vi "Prepare_TTL_activation_sequence.vi"(5 "Conditions presets array":T1 {"Specifier(s)"."Validity criteria(s)"."Validity value" min=0.0 step=0.1 format="%.2g"; "Specifier(s)"."Value" step=1.0 format="%#.2g"}, 7 "IO parameters.IO inversion config.":u16, 8 "Error In":errorcluster, 10 "Rules (conditions) became FALSE":bool[](array[boolean])=[FALSE, FALSE, FALSE, FALSE], 11 "Rules (conditions) became TRUE":bool[](array[boolean])=[FALSE, FALSE, FALSE, FALSE]) -> (0 "Error Out":errorcluster, 3 "TTL command(s) out":cluster{"Numeric":dbl, "String":string}[](array[cluster]))   [LabVIEW 2018, in "TTL IO.lvlib"]
uses:
  TTL IO.lvlib
  SubVi's/Controls/CTL_Conditions_Array.ctl
  SubVi's/Controls/CTL_Conditions_Cluster.ctl
  SubVi's/Controls/CTL_Condition_type.ctl
  SubVi's/Controls/CTL_Comparison_type.ctl
  SubVi's/Controls/CTL_Validity_check_criteria.ctl
  SubVi's/Controls/CTL_Response_info.ctl
  SubVi's/Controls/CTL_Condition_response_type.ctl
  SubVi's/Controls/CTL_Reponse_port_info.ctl
  <userlib>/_OpenG.lib/array/array.llb/Sort 1D Array (DBL)__ogtk.vi
  <userlib>/_OpenG.lib/array/array.llb/Reorder 1D Array2 (U8)__ogtk.vi
  <userlib>/_OpenG.lib/array/array.llb/Remove Duplicates from 1D Array (U8)__ogtk.vi
  <userlib>/_OpenG.lib/array/array.llb/Search 1D Array (DBL)__ogtk.vi
  <userlib>/_OpenG.lib/array/array.llb/Delete Elements from 1D Array (U8)__ogtk.vi
  <userlib>/_OpenG.lib/array/array.llb/Delete Elements from 1D Array (DBL)__ogtk.vi
  Tracker.lvlib
  Common_Resources.lvlib
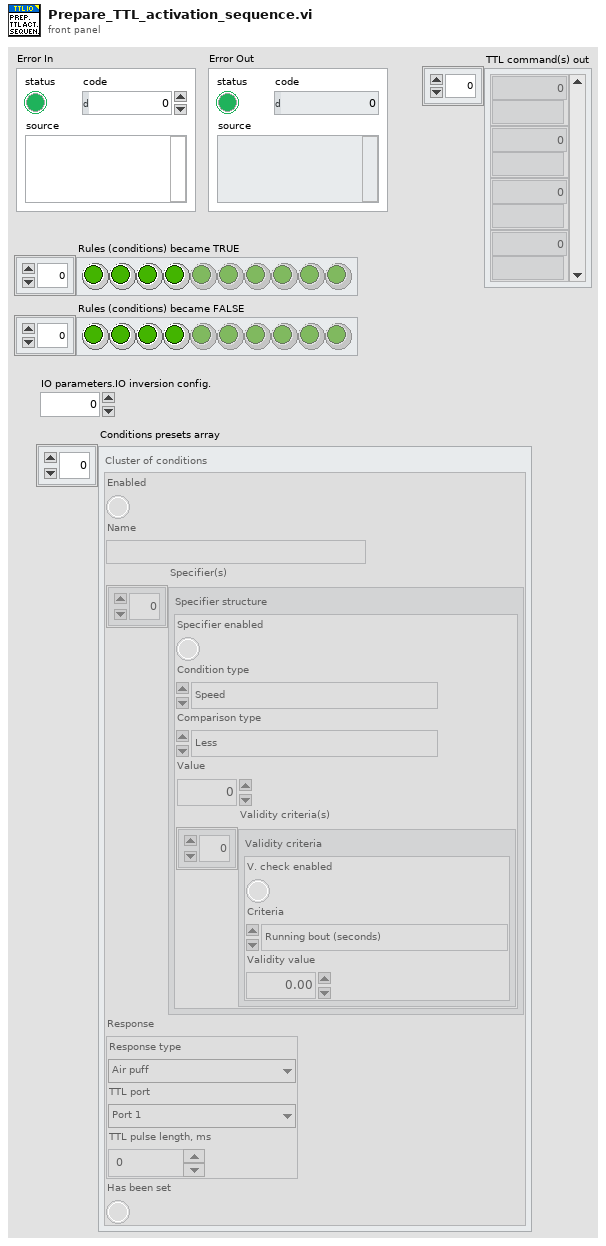
[diagram p1: front panel]
types:
  T1 = typedef "Common_Resources.lvlib/CTL_Conditions_Array.ctl" = T2[]
  T2 = typedef "Common_Resources.lvlib/CTL_Conditions_Cluster.ctl" = cluster{"Enabled":bool, "Name":string, "Specifier(s)":cluster{"Specifier enabled":bool, "Condition type":T3, "Comparison type":T4, "Value":dbl, "Validity criteria(s)":cluster{"V. check enabled":bool, "Criteria":T5, "Validity value":dbl}[]}[], "Response":T6, "Has been set":bool}
  T3 = typedef "Common_Resources.lvlib/CTL_Condition_type.ctl" = enum16{"Speed", "Zone", "Angle to wall"}
  T4 = typedef "Common_Resources.lvlib/CTL_Comparison_type.ctl" = enum16{"Less", "Less or Equal", "Equal", "Greater or Equal", "Greater", "Not Equal"}
  T5 = typedef "Common_Resources.lvlib/CTL_Validity_check_criteria.ctl" = enum16{"Running bout (seconds)", "Running bout (meters)"}
  T6 = typedef "Common_Resources.lvlib/CTL_Response_info.ctl" = cluster{"Response type":T7, "TTL port":T8, "TTL pulse length, ms":dbl}
  T7 = typedef "Common_Resources.lvlib/CTL_Condition_response_type.ctl" = enum16{"None", "Air puff", "Liquid reward"}
  T8 = typedef "Common_Resources.lvlib/CTL_Reponse_port_info.ctl" = enum16{"Port 1", "Port 2", "Port 3", "Port 4"}
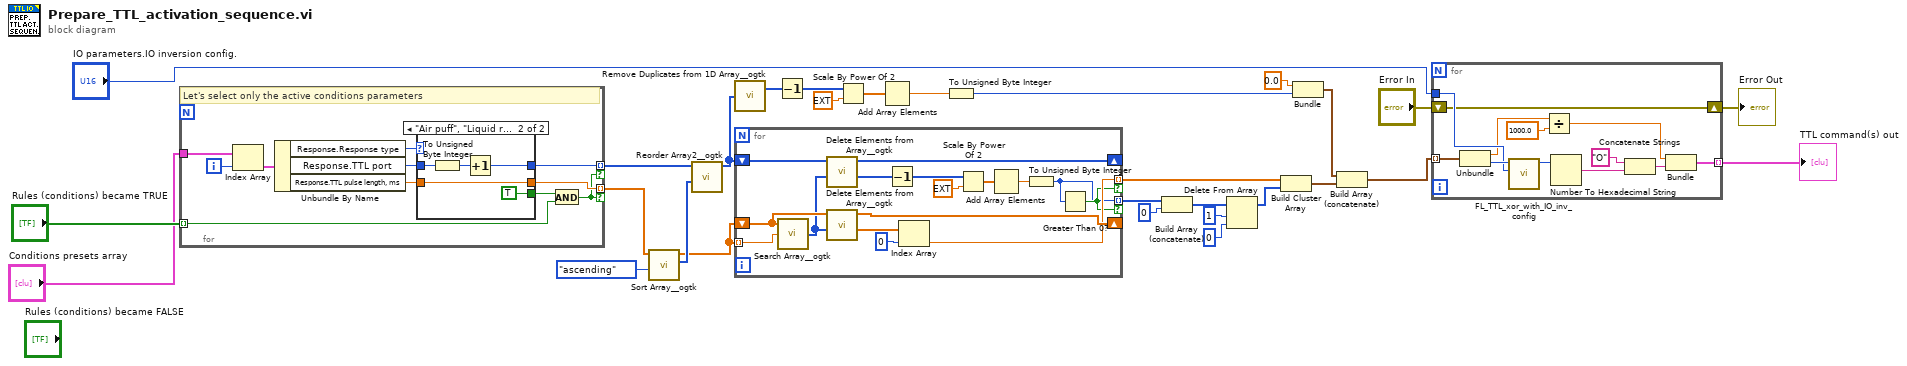
[diagram p0: block diagram]
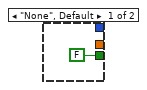
[diagram p2: hidden frame]
diagram:
  n1 = for {
    tunnel: "Rules (conditions) became TRUE" -> [w35] mode=indexing
    tunnel: "Conditions presets array" -> [w40]
    tunnel: [w32] -> w13 mode=indexing if=w30
    tunnel: [w31] -> w11 mode=indexing if=w30
    i -> [w33]
    # "Let's select only the active conditions parameters"
    n2 = Index Array(array=w40, index=w33) -> (element=w39:T2)
    n3 = Unbundle By Name(w39) -> ("Response.Response type"=w38:T7, "Response.TTL port"=w37:T8, "Response.TTL pulse length, ms"=w36:dbl)
    n4 = case shown="\"Air puff\", \"Liquid reward\"" w38 {
      tunnel: w37 -> [_ w43]
      tunnel: w36 -> [_ w45]
      tunnel: [FALSE TRUE] -> w34
      tunnel: [_ w45] -> w32
      tunnel: [_ w42] -> w31
      frame "None", Default {
      }
      frame "Air puff", "Liquid reward" {
        n5 = To Unsigned Byte Integer(number=w43) -> (unsigned 8bit integer=w44:u8)
        n6 = Increment(x=w44) -> (x+1=w42:u8)
      }
    }
    n7 = And(x=w34, y=w35) -> (x .and. y?=w30:bool)
  }
  n8 = call-poly <userlib>:"Sort Array__ogtk.vi"("Order"=enum16{"ascending", "descending"}."ascending", "Array in"=w13) -> ("Sorted Pointers"=w10:i32[], "Sorted Array out"=w9:dbl[])  [unwired: 8 in]
  n9 = call-poly <userlib>:"Reorder Array2__ogtk.vi"("indices"=w10, "array"=w11) -> ("reordered array"=w8:u8[])  [unwired: 9 in]
  n10 = call-poly <userlib>:"Remove Duplicates from 1D Array__ogtk.vi"("Input Array"=w8) -> ("Output Array"=w28:u8[])  [unwired: 1 out]
  n11 = for {
    tunnel: w9 -> [w62] mode=indexing
    shift-right: [w60] -> _
    shift-left: w9 -> [w61]
    shift-right: [w56] -> _
    shift-left: w8 -> [w58]
    tunnel: [w54] -> w21 mode=indexing if=w52
    tunnel: [w47] -> w26 mode=indexing if=w52
    n12 = call-poly <userlib>:"Search Array__ogtk.vi"("Array"=w61, "Element Data"=w62) -> ("Indices of Elements"=w57:i32[])  [unwired: 7 in]
    n13 = call-poly <userlib>:"Delete Elements from Array__ogtk.vi"("indices"=w57, "array"=w58) -> ("deleted elements"=w49:u8[], "array w/ subset deleted"=w56:u8[])  [unwired: 8 in]
    n14 = call-poly <userlib>:"Delete Elements from Array__ogtk.vi"("indices"=w57, "array"=w61) -> ("deleted elements"=w59:dbl[], "array w/ subset deleted"=w60:dbl[])  [unwired: 8 in]
    n15 = Decrement(x=w49) -> (x-1=w50:u8[])
    n16 = Index Array(array=w59, index=0) -> (element=w54:dbl)
    n17 = Scale By Power Of 2(n=w50, x=ext 1.0) -> (x*2^n=w48:ext[])
    n18 = Add Array Elements(numeric array=w48) -> (sum=w53:ext)
    n19 = To Unsigned Byte Integer(number=w53) -> (unsigned 8bit integer=w47:u8)
    n20 = Greater Than 0?(x=w47) -> (x > 0?=w52:bool)
  }
  n21 = Decrement(x=w28) -> (x-1=w4:u8[])
  n22 = Scale By Power Of 2(n=w4, x=ext 1.0) -> (x*2^n=w7:ext[])
  n23 = Add Array Elements(numeric array=w7) -> (sum=w14:ext)
  n24 = To Unsigned Byte Integer(number=w14) -> (unsigned 8bit integer=w5:u8)
  n25 = Build Array (concatenate)(w26, u8 0) -> (w24:u8[])
  n26 = Delete From Array(array=w24, length=1, index=0) -> (array with subset deleted=w3:u8[])  [unwired: 1 out]
  n27 = Build Cluster Array(w21, w3) -> (w20:cluster{dbl, u8}[])
  n28 = Bundle(0.0, w5) -> (w16:cluster{dbl, u8})  [unwired: 1 in]
  n29 = Build Array (concatenate)(w16, w20) -> (w17:cluster{dbl, u8}[])
  n30 = for {
    shift-right: [w68] -> w19
    shift-left: "Error In" -> [w68]
    tunnel: w17 -> [w74] mode=indexing
    tunnel: "IO parameters.IO inversion config." -> [w70]
    tunnel: [w63] -> w15 mode=indexing
    n31 = Unbundle(w74) -> (w66:dbl, w71:u8)
    n32 = call "FL_TTL_xor_with_IO_inv_config.vi"("IO inversion config."=w70, "TTL port(s) config to fire"=w71) -> ("ON config."=w69:u32)  [unwired: 8 in, 1 out]
    n33 = Divide(x=w66, y=1000.0) -> (x/y=w65:dbl)
    n34 = Number To Hexadecimal String(2:w69) -> (0:w73:string)  [unwired: 1 in]
    n35 = Concatenate Strings("O" ("string"), w73) -> (w67:string)
    n36 = Bundle(w65, w67) -> (w63:cluster{dbl, string})  [unwired: 1 in]
  }
  "Error Out" <- w19
  "TTL command(s) out" <- w15
